vi "pullObjFromAtlas.vi"(10 "slice":u32, 11 "Atlas":path) -> (3 "Array":sgl[](array[numeric]))   [LabVIEW 2013]
uses:
  imagereconstruction/x64/Debug/labviewdll.dll
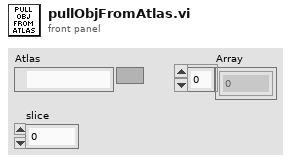
[diagram p1: front panel]
types:
  T1 = typedef "tags_cluster.ctl" = cluster{"compression":i32, "image width":i32, "image length":i32, "host computer":string, "software":string, "bitness":i32, "number of pages":i32, "samples per pixel":i32, "scanline size":i32, "strip size":i32, "lines per strip":i32}
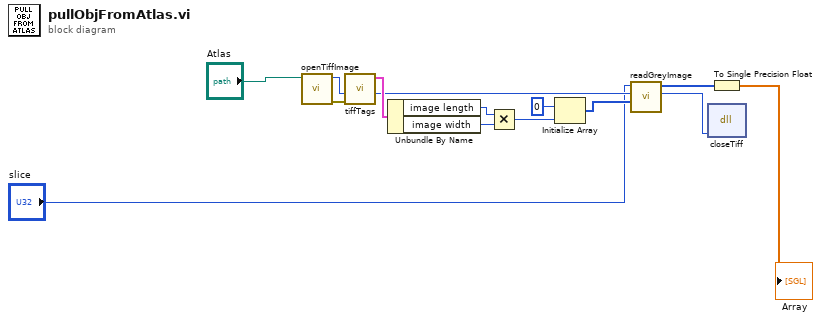
[diagram p0: block diagram]
diagram:
  n1 = call "openTiffImage.vi"("NewVal"="Atlas") -> ("error out"=w2:errorcluster, "returned pointer"=w1:i64)  [unwired: 9 in]
  n2 = call "tiffTags.vi"("error in (no error)"=w2, "tif pointer"=w1) -> ("tiff pointer"=w5:i64, "Image Properties"=w8:T1)  [unwired: 7 in, 1 out]
  n3 = Unbundle By Name(w8) -> ("image length"=w9:i32, "image width"=w10:i32)
  n4 = Multiply(x=w9, y=w10) -> (x*y=w11:i32)
  n5 = Initialize Array(u8 0 ("element"), w11) -> (w6:u8[])
  n6 = call "readGreyImage.vi"("raster"=w6, "tif"=w5, "Image Number"="slice") -> ("tif pointer"=w14:i64, "pixels"=w12:u8[])  [unwired: 5 in, 2 out]
  n7 = dll-call lib="D:/work/uni/FYP/reconrepo/imagereconstruction/x64/Debug/labviewdll.dll" fn="closeTiff"("tiff"=w14) -> ()  [unwired: 5 in, 2 out]
  n8 = To Single Precision Float(number=w12) -> (single precision float=→"Array":sgl[])
